vi "Dequeue and Write to CSV.vi"(0 "Queue name":string="Data", 1 "Queue data type":cluster{"Numeric":dbl, dbl, dbl, dbl, dbl}, 2 "Absolute file path of CSV":path=path "/home/lvuser", 3 "Error In":errorcluster, 4 "Record data":bool) -> (5 "error out":errorcluster)   [LabVIEW 2018]
uses:
  <vilib>/Utility/file.llb/Write Delimited Spreadsheet (DBL).vi
panel:
  out "Queue empty":bool
  in  "Stop":bool
  out "Elements in queue":i32(slide) scale=0.0..10.0
  out "Elements stored":i32(slide) scale=0.0..10.0
  # "INPUTS"
  # "PURPOSE\nThis VI dequeues elements from queue 'Queue name', and writes them to a CSV file in location 'Absolute file path of CSV'..\n\nUSE\nOpen the block diagram and verify the data type of the queue matches that of the portion of the calling VI that enqueues the data being dequeued by this VI. If it does not then adjust portions (1) and (2) of the block diagram accordingly."
  # "OUTPUTS"
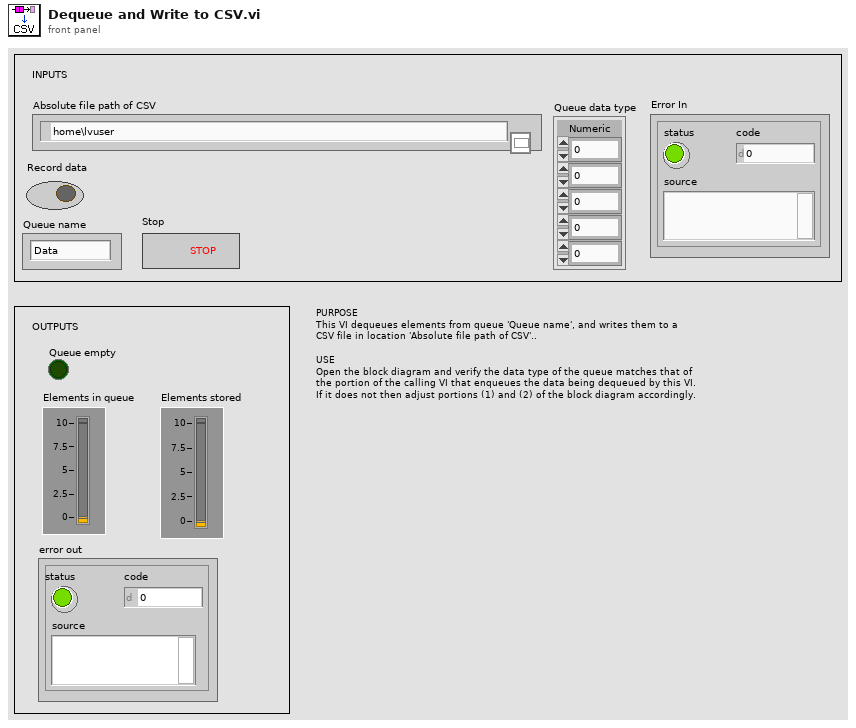
[diagram p1: front panel]
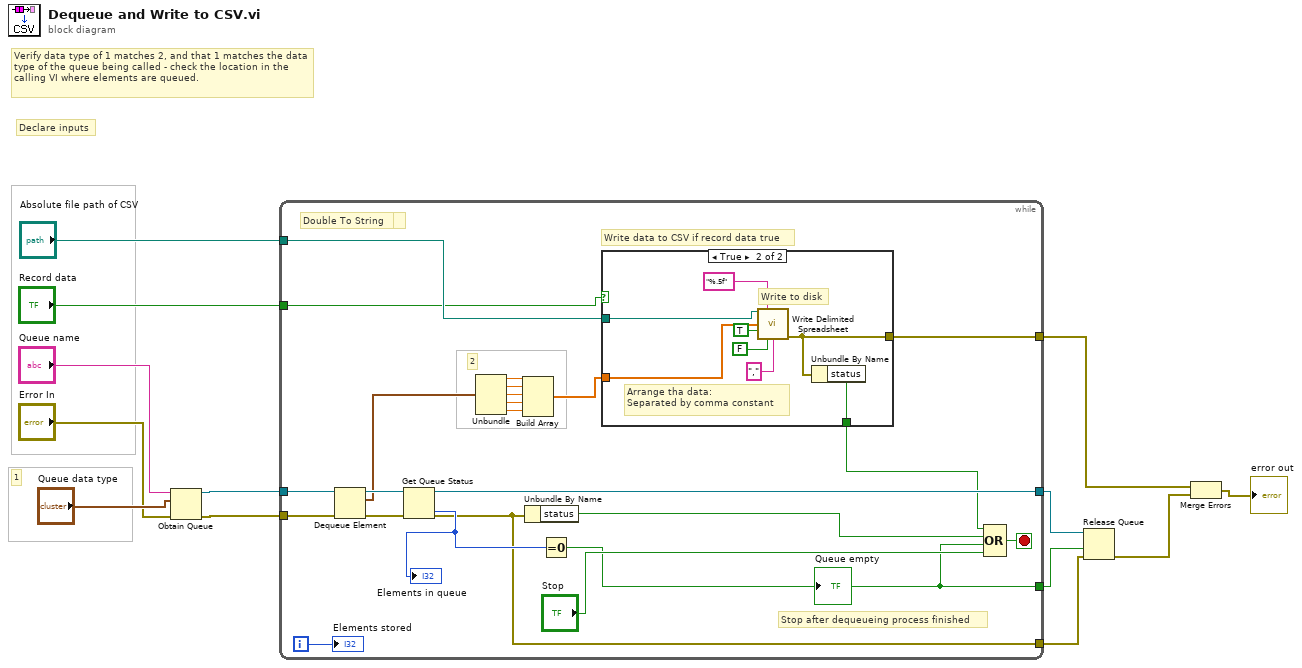
[diagram p0: block diagram]
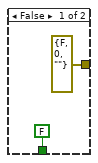
[diagram p2: hidden frame]
diagram:
  # "Declare inputs"
  # "1"
  # "Verify data type of 1 matches 2, and that 1 matches the data type of the queue being called - check the location in the calling VI where elements are queued."
  n1 = Obtain Queue(name (unnamed)="Queue name", element data type="Queue data type", error in (no error)="Error In") -> (queue out=w11:refnum<queue>, error out=w10:errorcluster)  [unwired: 2 in, 1 out]
  n2 = while {
    tunnel: w11 -> [w35]
    tunnel: [w31] -> w12
    tunnel: w10 -> [w28]
    tunnel: [w26] -> w8
    tunnel: "Absolute file path of CSV" -> [w24]
    tunnel: [w21] -> w3
    tunnel: "Record data" -> [w20]
    tunnel: [w14] -> w1
    i -> [w29]
    stop <- w36 stop-if-true
    # "Write data to CSV if record data true"
    # "2"
    # "Data Logging Loop"
    # "Stop after dequeueing process finished"
    # "Double To String"
    n3 = Dequeue Element(queue=w35, error in (no error)=w28) -> (queue out=w33:refnum<queue>, element=w27:cluster{"Numeric":dbl, dbl, dbl, dbl, dbl}, error out=w32:errorcluster)  [unwired: 1 in, 1 out]
    n4 = Get Queue Status(queue=w33, error in (no error)=w32) -> (queue out=w31:refnum<queue>, error out=w26:errorcluster, # elements in queue=w30:i32)  [unwired: 1 in, 5 out]
    "Elements in queue" <- w30
    n5 = Unbundle(w27) -> ("Numeric"=w19:dbl, w18:dbl, w17:dbl, w16:dbl, w15:dbl)
    n6 = Build Array(w19, w18, w17, w16, w15) -> (w23:dbl[])
    n7 = Unbundle By Name(w26) -> ("status"=w34:bool)
    n8 = Equal To 0?(x=w30) -> (x = 0?=w14:bool)
    "Queue empty" <- w14
    n9 = case shown="True" w20 {
      tunnel: w24 -> [_ w46]
      tunnel: w23 -> [_ w44]
      tunnel: [errorcluster {"status"=FALSE, "code"=0, "source"=""} ("error out") w40] -> w21
      tunnel: [FALSE ("status") w39] -> w22
      frame False {
      }
      frame True {
        # "Write to disk"
        # "Arrange tha data:\nSeparated by comma constant"
        n10 = call-poly <vilib>:"Write Delimited Spreadsheet.vi"("file path (dialog if empty)"=w46, "format (%.3f)"="%.5f", "1D data"=w44, "append to file? (new file:F)"=TRUE, "transpose? (no:F)"=FALSE, "delimiter (\\t)"="," ("delimiter (\\t)")) -> ("error out"=w40:errorcluster)  [unwired: 8 in, 1 out]
        n11 = Unbundle By Name(w40) -> ("status"=w39:bool)
      }
    }
    n12 = Compound Arithmetic op=OR(w22, w34, w14, "Stop") -> (w36:bool)
    "Elements stored" <- w29
  }
  n13 = Release Queue(queue=w12, force destroy? (F)=w1, error in (no error)=w8) -> (error out=w5:errorcluster)  [unwired: 2 out]
  n14 = Merge Errors(w3, w5) -> (→"error out":errorcluster)
